vi "TestDynamixelExploration.vi"() -> ()   [LabVIEW 2013]
doc: "Test that all hooked up Dynamixels move to desired position and can tell us their status.\n\nBe sure to set the serial port name before running!\n\nEric Schneider and Elizabeth Mahon, 4-7-2014"
uses:
  <instrlib>/Dynamixel Motor/Public/Motor Operation/Low Level/Baud Setting.ctl
  <vilib>/addons/control/pid/pid.llb/PID (DBL Array).vi
  <instrlib>/Dynamixel Motor/Dynamixel Motor.lvlib
  <vilib>/addons/control/pid/NI_PID_pid.lvlib
panel:
  in  "Desired Velocity":dbl[](array[numeric])
  out "Load/Torque %":sgl[](array[numeric])
  out "Voltage":sgl[](array[numeric])
  in  "Desired Position":dbl[](array[numeric])
  in  "stop":bool
  out "Positions":dbl[](array[numeric])
  in  "VISA resource name":refnum<visa-resource-name>
  out "Motors IDs Found":u8[](array[numeric])
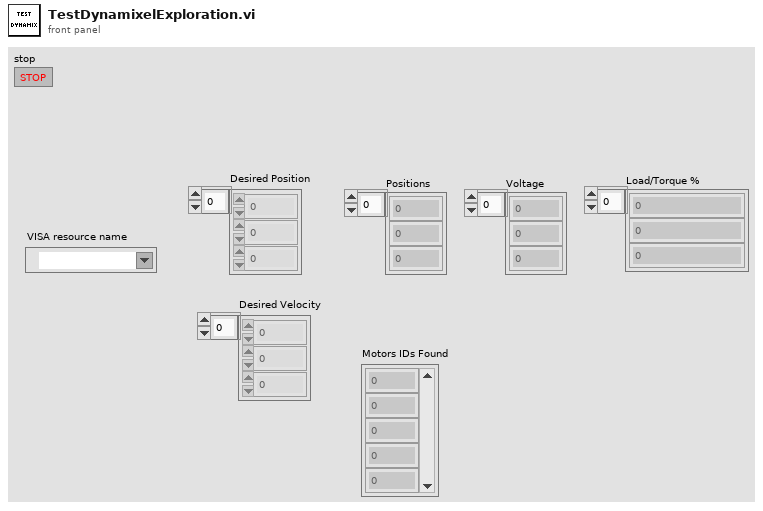
[diagram p1: front panel]
types:
  T1 = typedef "Dynamixel Motor.lvlib/Baud Setting.ctl" = u8
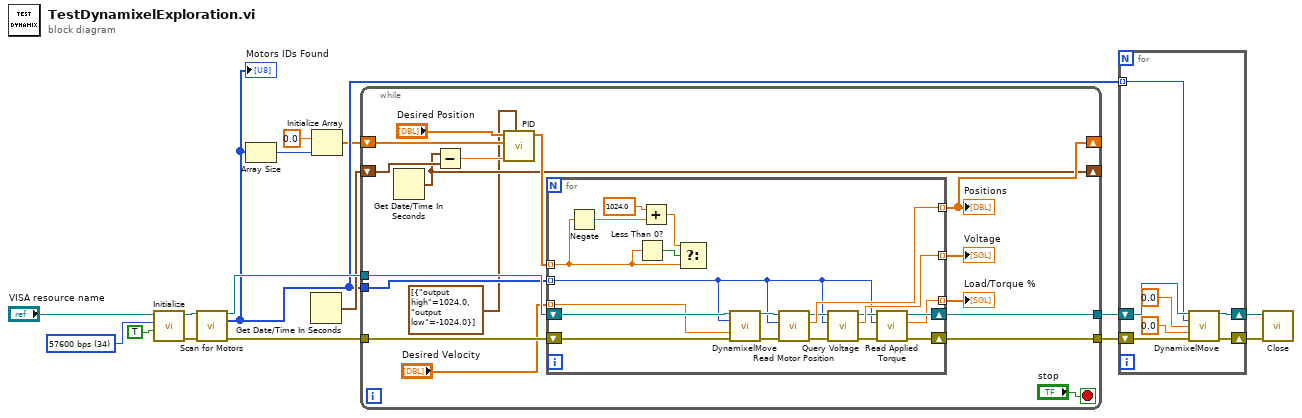
[diagram p0: block diagram]
diagram:
  w9 = T1 34 items=["1,000,000 bps"=1, "500,000 bps"=3, "400,000 bps"=4, "250,000 bps"=7, "200,000 bps"=9, "115200 bps"=16, "57600 bps"=34, "19200 bps"=103, "9600 bps"=207] ("Baud rate (57600 bps)")
  n1 = call <instrlib>:"Initialize.vi"("Force Baud Rate (True)"=TRUE, "Baud rate (57600 bps)"=w9, "VISA resource name"="VISA resource name") -> ("error out"=w10:errorcluster, "VISA resource name out"=w11:refnum<visa-resource-name>)  [unwired: 7 in]
  n2 = call <instrlib>:"Scan for Motors.vi"("VISA resource name"=w11, "error in (no error)"=w10) -> ("VISA resource name out"=w16:refnum<visa-resource-name>, "Motors IDs Found"=w3:u8[], "error out"=w15:errorcluster)  [unwired: 11 in]
  "Motors IDs Found" <- w3
  n3 = Array Size(array=w3) -> (size(s)=w4:i32)
  n4 = Get Date/Time In Seconds() -> (seconds since 1Jan1904=w5:timestamp)
  n5 = Initialize Array(0.0 ("element"), w4) -> (w1:dbl[])
  n6 = while {
    tunnel: w16 -> [w33]
    tunnel: w15 -> [w32]
    tunnel: [w31] -> w14
    tunnel: [w30] -> w13
    tunnel: w3 -> [w29]
    shift-right: [w23] -> _
    shift-left: w1 -> [w22]
    shift-right: [w20] -> _
    shift-left: w5 -> [w21]
    stop <- "stop" stop-if-true
    n7 = Get Date/Time In Seconds() -> (seconds since 1Jan1904=w20:timestamp)
    n8 = Subtract(x=w20, y=w21) -> (x-y=w19:dbl)
    n9 = call-poly <vilib>:"PID.vi"("output range"=cluster{"output high":dbl, "output low":dbl}[] [{"output high"=1024.0, "output low"=-1024.0}], "dt (s)"=w19, "process variable"=w22, "setpoint"="Desired Position") -> ("output"=w24:dbl[])  [unwired: 6 in, 1 out]
    n10 = for {
      tunnel: w29 -> [w41] mode=indexing
      shift-right: [w43] -> w31
      shift-left: w33 -> [w52]
      shift-right: [w42] -> w30
      shift-left: w32 -> [w51]
      tunnel: [w49] -> w23 mode=indexing
      tunnel: [w46] -> w27 mode=indexing
      tunnel: [w40] -> w26 mode=indexing
      tunnel: w24 -> [w38] mode=indexing
      tunnel: "Desired Velocity" -> [w34] mode=indexing
      n11 = Negate(x=w38) -> (-x=w36:dbl)
      n12 = Less Than 0?(x=w38) -> (x < 0?=w39:bool)
      n13 = Add(x=1024.0, y=w36) -> (x+y=w37:dbl)
      n14 = Select(t=w37, s=w39, f=w38) -> ()  [unwired: 1 out]
      n15 = call "DynamixelMove.vi"("VISA resource name"=w52, "Motor ID (0)"=w41, "Goal Speed (RPM)"=w34, "error in (no error)"=w51) -> ("VISA resource name out"=w53:refnum<visa-resource-name>, "error out"=w50:errorcluster)  [unwired: 10 in]
      n16 = call <instrlib>:"Read Motor Position.vi"("error in (no error)"=w50, "Motor ID (0)"=w41, "VISA resource name"=w53) -> ("error out"=w48:errorcluster, "Position (deg)"=w49:dbl, "VISA resource name out"=w47:refnum<visa-resource-name>)  [unwired: 6 in]
      n17 = call <instrlib>:"Query Voltage.vi"("error in (no error)"=w48, "Motor ID (0)"=w41, "VISA resource name"=w47) -> ("error out"=w45:errorcluster, "Voltage (V)"=w46:sgl, "VISA resource name out"=w44:refnum<visa-resource-name>)  [unwired: 6 in]
      n18 = call <instrlib>:"Read Applied Torque.vi"("error in (no error)"=w45, "Motor ID (0)"=w41, "VISA resource name"=w44) -> ("error out"=w42:errorcluster, "Load/torque %"=w40:sgl, "VISA resource name out"=w43:refnum<visa-resource-name>)  [unwired: 6 in]
    }
    "Positions" <- w23
    "Voltage" <- w27
    "Load/Torque %" <- w26
  }
  n19 = for {
    shift-right: [w57] -> w7
    shift-left: w14 -> [w56]
    shift-right: [w58] -> w6
    shift-left: w13 -> [w55]
    tunnel: w3 -> [w54] mode=indexing
    n20 = call "DynamixelMove.vi"("VISA resource name"=w56, "Motor ID (0)"=w54, "Goal Position (150 deg)"=0.0, "Goal Speed (RPM)"=0.0, "error in (no error)"=w55) -> ("VISA resource name out"=w57:refnum<visa-resource-name>, "error out"=w58:errorcluster)  [unwired: 9 in]
  }
  n21 = call <instrlib>:"Close.vi"("error in (no error)"=w6, "VISA resource name"=w7) -> ()  [unwired: 9 in, 1 out]
